vi "ClockSelection1212.vi"(0 "FPGA Interface In":refnum<k20>, 1 "INTERNAL CLOCK":u8(ring) items=["From Oscillator", "From FPGA Clock"], 2 "CLOCK SELECTION":u8(ring) items=["Internal", "External (From SMA)"], 3 "error in (no error)":errorcluster, 4 "RIO Device":T1) -> (5 "FPGA Interface Out":refnum<k20>, 6 "RIO Device out":T1, 7 "error out":errorcluster)   [LabVIEW 2018]
uses:
  <vilib>/userdefined/High Color/nirio_resource_hc.ctl
  <vilib>/LabVIEW Targets/FPGA/FlexRIO/CustomFPGAMethods/79XXR_Method_IOModuleStatusImpl.vi
  <vilib>/Utility/error.llb/Error Cluster From Error Code.vi
  <vilib>/rvi/errors/niLvFpgaAdjustHostInterfaceError.vi
  <vilib>/FPGAPlugInAG/Dynamic/niLvFpga_Close_Dynamic.vi
  <vilib>/rvi/interface/nirviMethod/nirviMethod.xnode
  <vilib>/rvi/interface/nirviReadWriteControl/nirviReadWriteControl.xnode
  <vilib>/rvi/interface/nirviCloseFPGA/nirviCloseFPGA.xnode
  NiFpgaLv.dll
  <vilib>/rvi/interface/Simulation/niFpgaSimulationCallBeginRW.vi
panel:
  out "IO Enabled? 2":bool
  out "TimeOut?":bool
  out "IO Enabled?":bool
  in  "DEBUG":bool
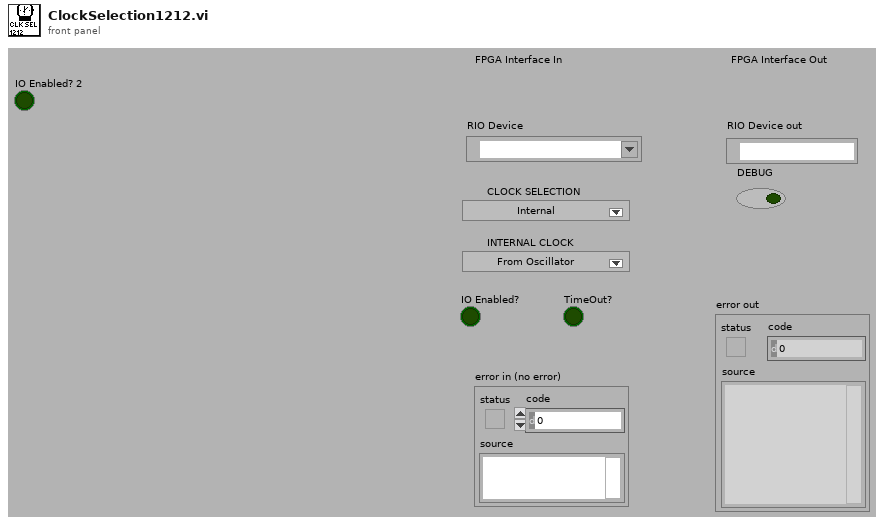
[diagram p1: front panel]
types:
  T1 = typedef "nirio_resource_hc.ctl" = tag
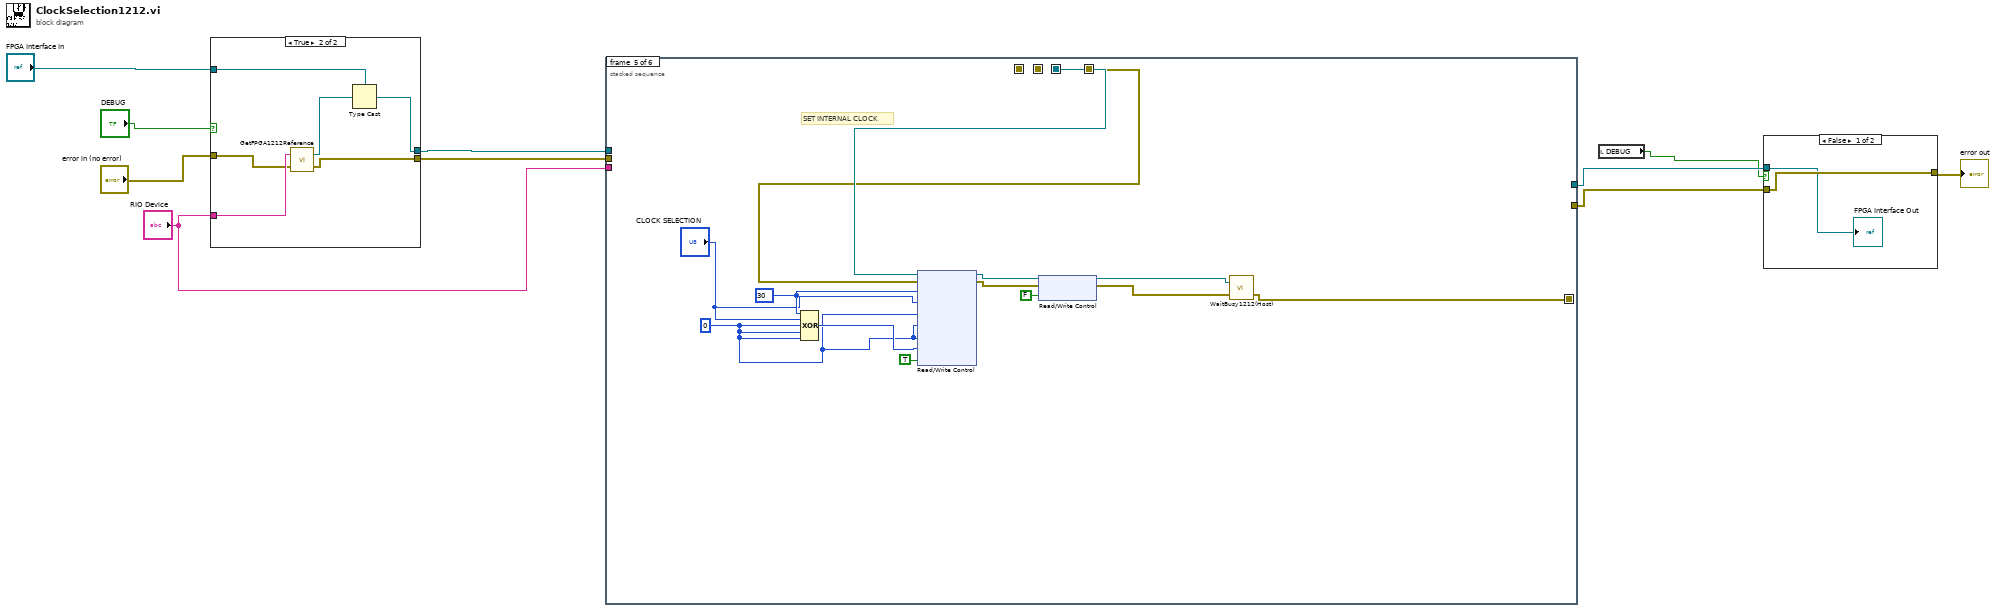
[diagram p0: block diagram]
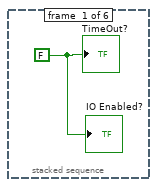
[diagram p2: hidden frame]
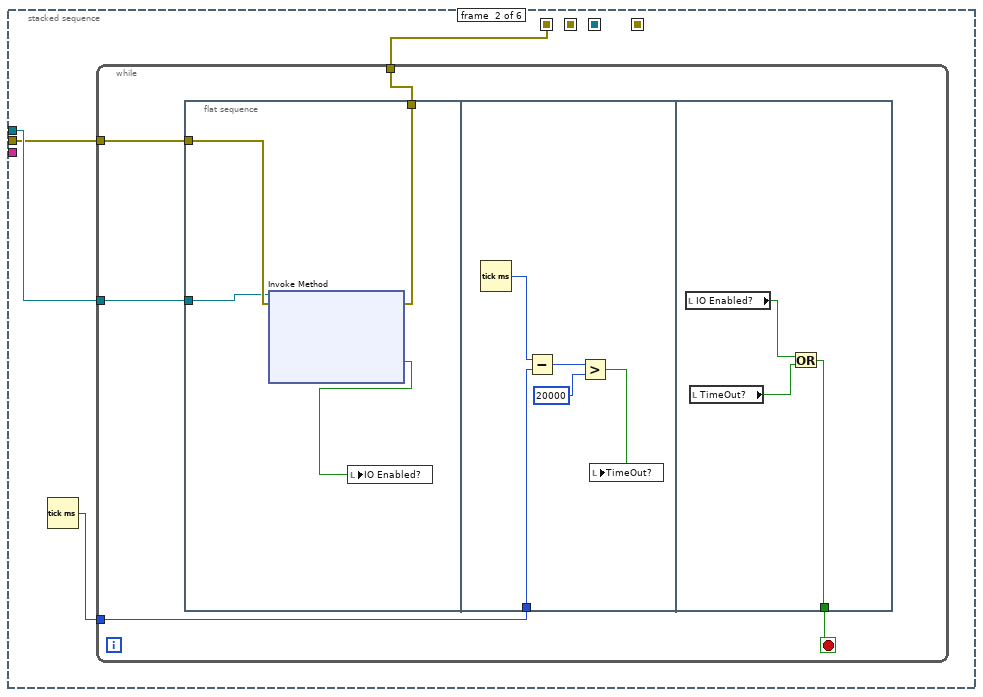
[diagram p3: hidden frame]
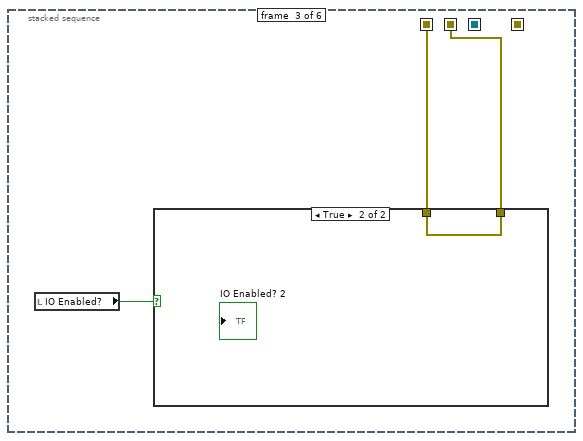
[diagram p4: hidden frame]
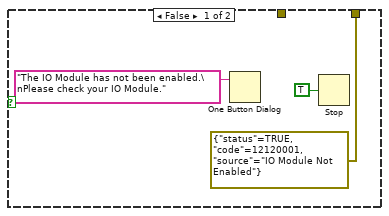
[diagram p5: hidden frame]
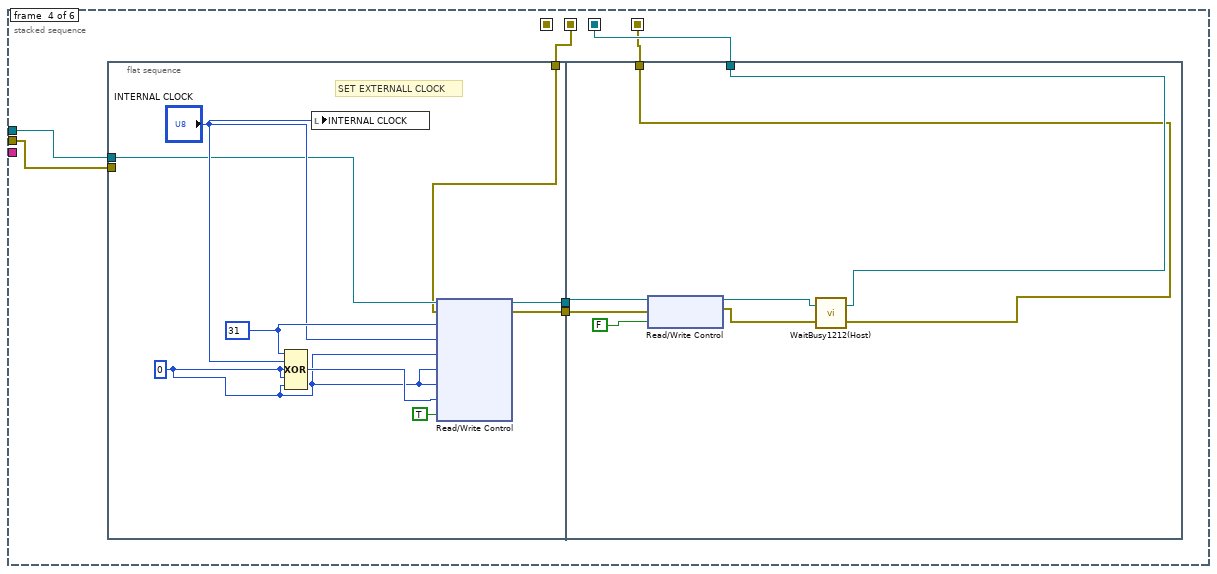
[diagram p6: hidden frame]
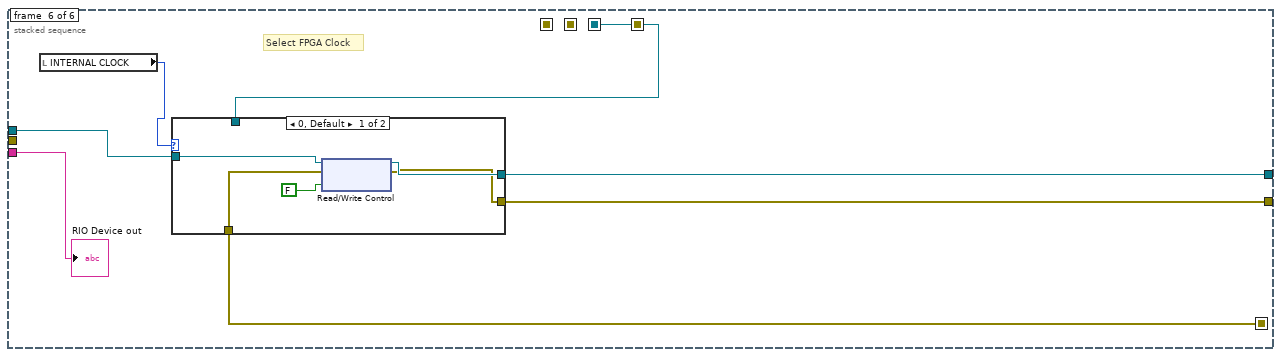
[diagram p7: hidden frame]
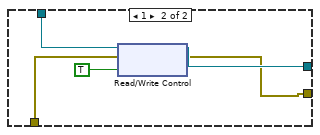
[diagram p8: hidden frame]
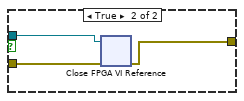
[diagram p9: hidden frame]
diagram:
  n1 = case shown="True" "DEBUG" {
    tunnel: "RIO Device" -> [_ w16]
    tunnel: "error in (no error)" -> [w12 w15]
    tunnel: [w12 w13] -> w5
    tunnel: [w11 w17] -> w3
    tunnel: "FPGA Interface In" -> [w11 w18]
    frame False {
    }
    frame True {
      n2 = call "GetFPGA1212Reference.vi"("error in"=w15, "RIO Device IN"=w16) -> ("error out"=w13:errorcluster, "FPGA VI Reference Out"=w14:refnum<k20>)
      n3 = Type Cast(type=w18, x=w14) -> (*(type *) &x=w17:refnum<k20>)
    }
  }
  n4 = stacked-sequence {
    seq-local: [_ _ _ _ w71 _] -> [_ _ _ _ _ w85]
    seq-local: [_ _ _ w51 _ _] -> [_ _ _ _ w75 _]
    seq-local: [_ _ _ w52 _ _] -> [_ _ _ _ w76 w89]
    seq-local: [_ w20 _ _ _ _] -> [_ _ w41 _ _ _]
    seq-local: [_ _ w42 _ _ _] -> [_ _ _ w48 _ _]
    tunnel: "RIO Device" -> [_ _ _ _ _ w84]
    tunnel: w5 -> [_ w21 _ w54 _ _]
    tunnel: [_ _ _ _ _ w88] -> w7
    tunnel: [_ _ _ _ _ w90] -> w4
    tunnel: w3 -> [_ w23 _ w53 _ w87]
    frame #0 {
      w19 = FALSE ("TimeOut?")
      "TimeOut?" <- w19
      "IO Enabled?" <- w19
    }
    frame #1 {
      n5 = Tick Count (ms)() -> (millisecond timer value=w22:u32)
      n6 = while {
        tunnel: w23 -> [w28]
        tunnel: w22 -> [w27]
        tunnel: w21 -> [w25]
        tunnel: [w24] -> w20
        stop <- w26 stop-if-true
        n7 = flat-sequence {
          tunnel: w28 -> [w30]
          tunnel: w25 -> [w32]
          tunnel: [w31] -> w24
          tunnel: w27 -> [w34]
          tunnel: [w38] -> w26
          frame #0 {
            n8 = xnode "Invoke Method"("FPGA VI Reference In"=w30, "error in"=w32) -> ("error out"=w31:errorcluster, "IO Enabled?"=w29:bool)  [unwired: 4 out]
            n9 = local write "IO Enabled?"(w29) -> ()
          }
          frame #1 {
            n10 = Tick Count (ms)() -> (millisecond timer value=w37:u32)
            n11 = Subtract(x=w37, y=w34) -> (x-y=w36:u32)
            n12 = Greater?(x=w36, y=u32 20000) -> (0:w33:bool)
            n13 = local write "TimeOut?"(w33) -> ()
          }
          frame #2 {
            n14 = local read "IO Enabled?"() -> (w40:bool)
            n15 = local read "TimeOut?"() -> (w39:bool)
            n16 = Or(x=w40, y=w39) -> (x .or. y?=w38:bool)
          }
        }
      }
    }
    frame #2 {
      n17 = local read "IO Enabled?"() -> (w43:bool)
      n18 = case shown="True" w43 {
        tunnel: [errorcluster {"status"=TRUE, "code"=12120001, "source"="IO Module Not Enabled"} ("error out") w47] -> w42
        tunnel: w41 -> [_ w47]
        frame False {
          n19 = One Button Dialog(message="The IO Module has not been enabled.\nPlease check your IO Module.") -> ()  [unwired: 1 in, 1 out]
          n20 = Stop(stop? (T)=TRUE) -> ()
        }
        frame True {
        }
      }
    }
    frame #3 {
      n21 = flat-sequence {
        tunnel: w54 -> [_]
        tunnel: w53 -> [w59]
        tunnel: [w57] -> w50
        tunnel: [w56] -> w49
        tunnel: w48 -> [w55]
        tunnel: w50 -> [w69]
        tunnel: w49 -> [w68]
        tunnel: [w65] -> w52
        tunnel: [w64] -> w51
        frame #0 {
          w60 = u8 0
          w63 = u8 31 ("value")
          # "SET EXTERNALL CLOCK"
          n22 = Compound Arithmetic op=XOR(w63, "INTERNAL CLOCK", w60, w60, w60) -> (w62:u8)
          n23 = local write "INTERNAL CLOCK"("INTERNAL CLOCK") -> ()
          n24 = xnode "Read/Write Control"("FPGA VI Reference In"=w59, "error in"=w55, "DataI2c0"=w63, "DataI2c1"="INTERNAL CLOCK", "DataI2c2"=w60, "DataI2c3"=w60, "DataI2c4"=w60, "DataI2c5"=w62, "StartWRI2c"=TRUE) -> ("FPGA VI Reference Out"=w57:refnum<k20>, "error out"=w56:errorcluster)
        }
        frame #1 {
          n25 = xnode "Read/Write Control"("FPGA VI Reference In"=w69, "error in"=w68, "StartWRI2c"=FALSE) -> ("FPGA VI Reference Out"=w67:refnum<k20>, "error out"=w66:errorcluster)
          n26 = call "WaitBusy1212(Host).vi"("error in"=w66, "FPGA VI Reference In"=w67) -> ("error out"=w64:errorcluster, "FPGA VI Reference Out"=w65:refnum<k20>)
        }
      }
    }
    frame #4 {
      w80 = u8 0
      w82 = u8 30 ("value")
      # "SET INTERNAL CLOCK"
      n27 = Compound Arithmetic op=XOR(w82, "CLOCK SELECTION", w80, w80, w80) -> (w81:u8)
      n28 = xnode "Read/Write Control"("FPGA VI Reference In"=w76, "error in"=w75, "DataI2c0"=w82, "DataI2c1"="CLOCK SELECTION", "DataI2c2"=w80, "DataI2c3"=w80, "DataI2c4"=w80, "DataI2c5"=w81, "StartWRI2c"=TRUE ("IO Module\\starwri2c")) -> ("FPGA VI Reference Out"=w78:refnum<k20>, "error out"=w77:errorcluster)
      n29 = xnode "Read/Write Control"("FPGA VI Reference In"=w78, "error in"=w77, "StartWRI2c"=FALSE) -> ("FPGA VI Reference Out"=w73:refnum<k20>, "error out"=w72:errorcluster)
      n30 = call "WaitBusy1212(Host).vi"("error in"=w72, "FPGA VI Reference In"=w73) -> ("error out"=w71:errorcluster)  [unwired: 1 out]
    }
    frame #5 {
      # "Select FPGA Clock"
      n31 = local read "INTERNAL CLOCK"() -> (w86:u8)
      n32 = case shown="0, Default" w86 {
        tunnel: [w94 w100] -> w90
        tunnel: w89 -> [_ w97]
        tunnel: [w93 w99] -> w88
        tunnel: w87 -> [w95 _]
        tunnel: w85 -> [w91 w96]
        frame 0, Default {
          n33 = xnode "Read/Write Control"("FPGA VI Reference In"=w95, "error in"=w91, "Clock SEL"=FALSE) -> ("FPGA VI Reference Out"=w94:refnum<k20>, "error out"=w93:errorcluster)
        }
        frame 1 {
          n34 = xnode "Read/Write Control"("FPGA VI Reference In"=w97, "error in"=w96, "Clock SEL"=TRUE) -> ("FPGA VI Reference Out"=w100:refnum<k20>, "error out"=w99:errorcluster)
        }
      }
      "RIO Device out" <- w84
    }
  }
  n35 = local read "DEBUG"() -> (w2:bool)
  n36 = case shown="False" w2 {
    tunnel: [w102 w105] -> w8
    tunnel: w7 -> [w102 w104]
    tunnel: w4 -> [w101 w103]
    frame False {
      "FPGA Interface Out" <- w101
    }
    frame True {
      n37 = xnode "Close FPGA VI Reference"("FPGA VI Reference In"=w103, "error in"=w104) -> ("error out"=w105:errorcluster)
    }
  }
  "error out" <- w8
